vi "Query Bandwidth Part.vi"(0 "VISA resource name":refnum<visa-resource-name>, 5 "Instance (1)":T2=1, 7 "CC (1)":T1=1, 9 "BWP (BWP0)":i32(ring) items=["BWP0"], 11 "error in (no error)":errorcluster) -> (4 "VISA resource name out":refnum<visa-resource-name>, 6 "Subcarrier Spacing":i32, 8 "Cyclic Prefix":i32, 10 "No Of RBs":i32, 14 "Start RB":i32, 15 "error out":errorcluster)   [LabVIEW 2020, in "Rohde&Schwarz CMWXP NR FR1 Measurement.lvlib"]
doc: "Queries basic properties of the <BWP> on carrier <CC>.\n\nAttribute:\n-\n\nRemote-control command:\nCONFigure:NRSub:MEAS<i>[:CC<no>]:BWPart?"
uses:
  <instrlib>/Rohde&Schwarz CMWXP NR FR1 Measurement/Rohde&Schwarz CMWXP NR FR1 Measurement.lvlib
  <instrlib>/Rohde&Schwarz CMWXP NR FR1 Measurement/Private/_Instance.ctl
  <instrlib>/Rohde&Schwarz CMWXP NR FR1 Measurement/Private/_Carrier Component.ctl
  <instrlib>/Rohde&Schwarz CMWXP NR FR1 Measurement/Private/rsidr_core.llb/rsidr_core.lvlib
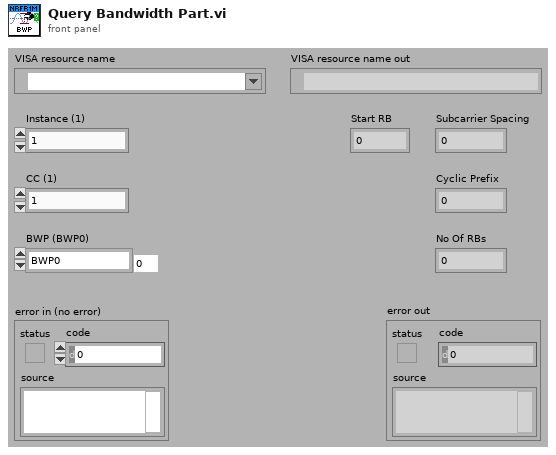
[diagram p1: front panel]
types:
  T1 = typedef "Rohde&Schwarz CMWXP NR FR1 Measurement.lvlib/_Carrier Component.ctl" = i32
  T2 = typedef "Rohde&Schwarz CMWXP NR FR1 Measurement.lvlib/_Instance.ctl" = i32
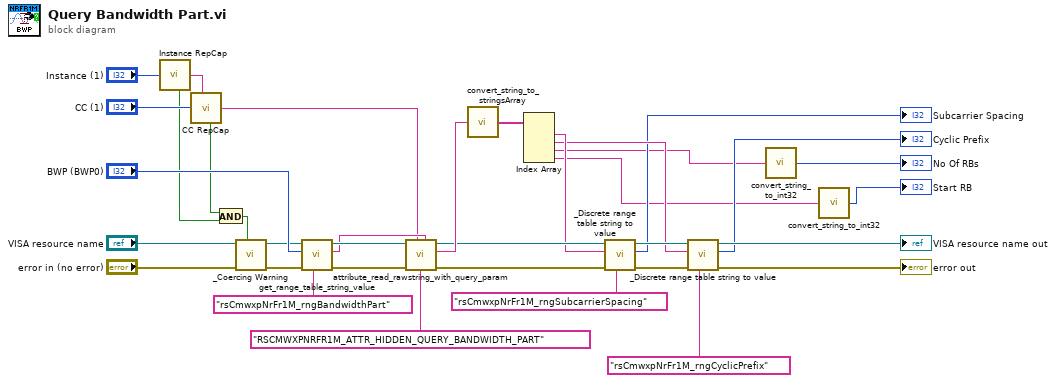
[diagram p0: block diagram]
diagram:
  n1 = call <instrlib>:"Instance RepCap.vi"("Instance In"="Instance (1)") -> ("In Range?"=w2:bool, "RepCap Identifier Out"=w34:string)  [unwired: 1 in]
  n2 = call <instrlib>:"CC RepCap.vi"("CC In"="CC (1)", "RepCap String In (\"\")"=w34) -> ("In Range?"=w1:bool, "RepCap Identifier Out"=w27:string)
  n3 = And(x=w1, y=w2) -> (x .and. y?=w3:bool)
  n4 = call <instrlib>:"_Coercing Warning.vi"("In Range?"=w3, "error in (no error)"="error in (no error)", "VISA resource name"="VISA resource name") -> ("error out"=w5:errorcluster, "VISA resource name out"=w4:refnum<visa-resource-name>)  [unwired: 7 in]
  n5 = call <instrlib>:"get_range_table_string_value.vi"("Range Table ID in"="rsCmwxpNrFr1M_rngBandwidthPart", "error in"=w5, "I32 input"="BWP (BWP0)", "VISA resource name"=w4) -> ("error out"=w30:errorcluster, "String Value out"=w28:string, "VISA resource name out"=w29:refnum<visa-resource-name>)  [unwired: 5 in]
  n6 = call <instrlib>:"attribute_read_rawstring_with_query_param.vi"("Query Parameter (None)"=w28, "Repeated Capability"=w27, "error in"=w30, "Attribute ID"="RSCMWXPNRFR1M_ATTR_HIDDEN_QUERY_BANDWIDTH_PART", "VISA resource name"=w29) -> ("error out"=w23:errorcluster, "Raw String out"=w25:string, "VISA resource name out"=w22:refnum<visa-resource-name>)  [unwired: 4 in]
  n7 = call <instrlib>:"convert_string_to_stringsArray.vi"("String in"=w25) -> ("string array out"=w24:string[])  [unwired: 3 in, 1 out]
  n8 = Index Array(array=w24) -> (element #1=w17:string, element #2=w16:string, element #3=w11:string, element #4=w9:string)  [unwired: 4 in]
  n9 = call <instrlib>:"_Discrete range table string to value.vi"("Discrete Range Table Identifier"="rsCmwxpNrFr1M_rngSubcarrierSpacing", "error in (no error)"=w23, "String Value In"=w17, "VISA resource name"=w22) -> ("error out"=w21:errorcluster, "Enum Value"=→"Subcarrier Spacing":i32, "VISA resource name out"=w20:refnum<visa-resource-name>)  [unwired: 5 in]
  n10 = call <instrlib>:"_Discrete range table string to value.vi"("Discrete Range Table Identifier"="rsCmwxpNrFr1M_rngCyclicPrefix", "error in (no error)"=w21, "String Value In"=w16, "VISA resource name"=w20) -> ("error out"=→"error out":errorcluster, "Enum Value"=→"Cyclic Prefix":i32, "VISA resource name out"=→"VISA resource name out":refnum<visa-resource-name>)  [unwired: 5 in]
  n11 = call <instrlib>:"convert_string_to_int32.vi"("String in"=w11) -> ("int32 value out"=→"No Of RBs":i32)  [unwired: 4 in]
  n12 = call <instrlib>:"convert_string_to_int32.vi"("String in"=w9) -> ("int32 value out"=→"Start RB":i32)  [unwired: 4 in]
